vi "FindLocalizedString.vi"(10 "LocalizationFileContent":T1, 11 "String[in]":string) -> (2 "Found":bool, 3 "LocalizedString":string)   [LabVIEW 2013]
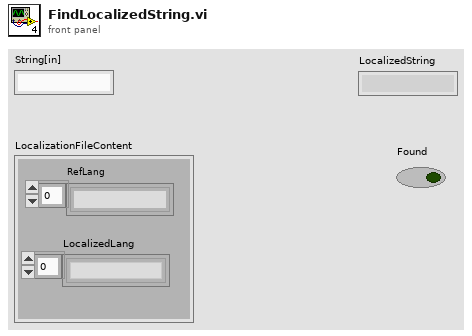
[diagram p1: front panel]
types:
  T1 = cluster{"RefLang":string[], "LocalizedLang":string[]}
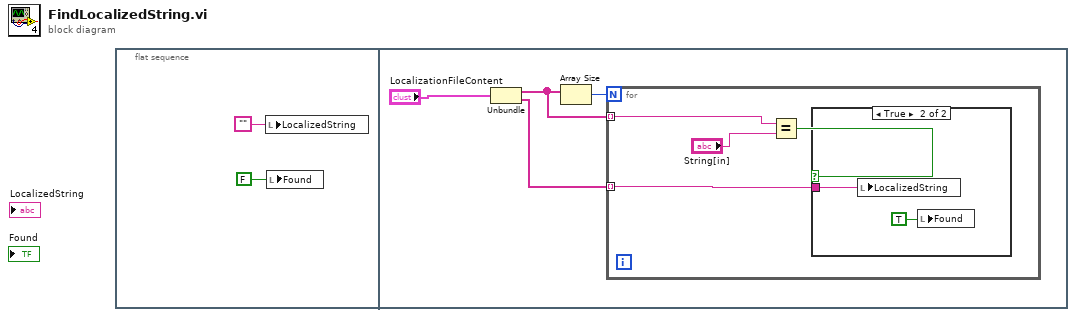
[diagram p0: block diagram]
diagram:
  n1 = flat-sequence {
    frame #0 {
      n2 = local write "LocalizedString"("") -> ()
      n3 = local write "Found"(FALSE) -> ()
    }
    frame #1 {
      n4 = Unbundle("LocalizationFileContent") -> ("RefLang"=w4:string[], "LocalizedLang"=w3:string[])
      n5 = Array Size(array=w4) -> (size(s)=w6:i32)
      n6 = for {
        N: w6 -> [_]
        tunnel: w4 -> [w8] mode=indexing
        tunnel: w3 -> [w7] mode=indexing
        n7 = Equal?(x=w8, y="String[in]") -> (x = y?=w10:bool)
        n8 = case shown="True" w10 {
          tunnel: w7 -> [_ w12]
          frame False {
          }
          frame True {
            n9 = local write "LocalizedString"(w12) -> ()
            n10 = local write "Found"(TRUE) -> ()
          }
        }
      }
    }
  }
